vi "RT Driver VI.vi"(6 "Device Clock":string, 9 "Device Inputs FIFO":refnum<k33>, 10 "Device Outputs FIFO":refnum<k33>, 11 "Device Reference":T1 format="%.0x") -> ()   [LabVIEW 2020, in "Routing and Faulting Engine.lvlib"]
uses:
  Routing and Faulting Engine.lvlib
  <vilib>/NI VeriStand/Custom Device API/Custom Device Item Ref.ctl
  <vilib>/NI VeriStand/Custom Device Tools/Custom Device Utility Library/Custom Device Utility Library.lvlib
  <vilib>/NI VeriStand/Custom Device API/Custom Device API.lvlib
panel:
  in  "Initialization Status Notifier":refnum<notifier>
  in  "Status Notifier":refnum<notifier>
  # "Custom Device Template\nv1.0"
  # "Use this template as a starting point for creating a custom device code module. The input controls shown here are specially named controls that the system will use to provide the device loop with data. The controls are not required for the device loop to run. For instance, if the device doesn't produce any output data, then you don't need the Device Outputs FIFO control. If you do use these controls, however, they need to have these exact names to be functional."
  # "The optional status notifier element is used to notify the RT engine of the last state of the custom device, and to indicate the device has completed execution. If this control is not used, a default No Error value is returned to the system when the device finishes execution.\n\nNote: This error state is not checked until the system shuts down. Use an output status channel to send more immediate status values to the system."
  # "This optional input can be used to send the VeriStand Engine the final status of the custom device initalization process. If this control exists on the custom device front panel, the VeriStand Engine will wait for a status update before starting up. If the custom device reports an error, that will abort the execution of the current configuration in the VeriStand Engine.\n\nThis control can be deleted if the custom device does not need to send the initialization status update."
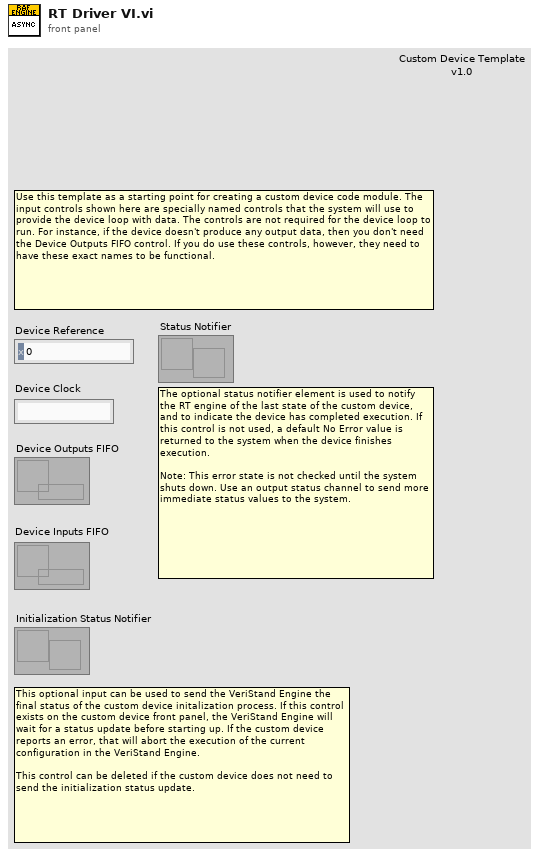
[diagram p1: front panel]
types:
  T1 = typedef "Custom Device API.lvlib/Custom Device Item Ref.ctl" = u64
  T2 = typedef "Custom Device API.lvlib/Custom Device Engine Event Ref.ctl" = refnum<event-registration>
  T3 = typedef "Routing and Faulting Engine.lvlib/Engine Data.ctl" = cluster{"Compiled.Settings":T4, "Producer":refnum<class "Abstract Producer.lvclass">, "Device Inputs":T13, "Device Outputs":T14, "States Changed":bool[]}
  T4 = typedef "Routing and Faulting Shared.lvlib/Compiled.Settings.ctl" = cluster{"Custom Device Name":string, "Communication Configuration":T5, "Routing and Faulting Configuration":T6, "Status Channels FIFO Indices":T12}
  T5 = typedef "Routing and Faulting Shared.lvlib/Communication Configuration.ctl" = cluster{"Consumer Queue Names":string[]}
  T6 = typedef "Routing and Faulting Shared.lvlib/Routing and Faulting Configuration.ctl" = cluster{"Routing Channel Configurations":T7[], "Alias Mappings":T9[], "Compiled Connection Buffer":T11[], "Compiled Initial Connection Indices":i32[]}
  T7 = typedef "Routing and Faulting Shared.lvlib/Routing Channel Configuration.ctl" = cluster{"Channel Name":string, "Initial Value":dbl, "FIFO Index":i32, "Value-Connections Map":T8}
  T8 = typedef "Routing and Faulting Shared.lvlib/Value-Connections Map.ctl" = cluster{"State Value Array":i32[], "Connection List Array":cluster{"Compiled Connections Indices":i32[]}[]}
  T9 = typedef "Routing and Faulting Shared.lvlib/Alias Mapping.ctl" = cluster{"Alias":string, "Endpoint":T10}
  T10 = typedef "Routing and Faulting Shared.lvlib/Alias Endpoint.ctl" = cluster{"Module Path":string, "Endpoint":string}
  T11 = typedef "Routing and Faulting Shared.lvlib/Compiled Connection.ctl" = cluster{"Consumer Queue Index":i32, "Normalized Connection String":string}
  T12 = typedef "Routing and Faulting Shared.lvlib/FIFO Indices.ctl" = cluster{"Status Channel":i32, "Heartbeat Channel":i32}
  T13 = typedef "Routing and Faulting Engine.lvlib/Device Inputs.ctl" = cluster{"Current Inputs":dbl[], "Previous Inputs":dbl[], "Device Inputs FIFO":refnum<k33>}
  T14 = typedef "Routing and Faulting Engine.lvlib/Device Outputs.ctl" = cluster{"Outputs":dbl[], "Device Outputs FIFO":refnum<k33>}
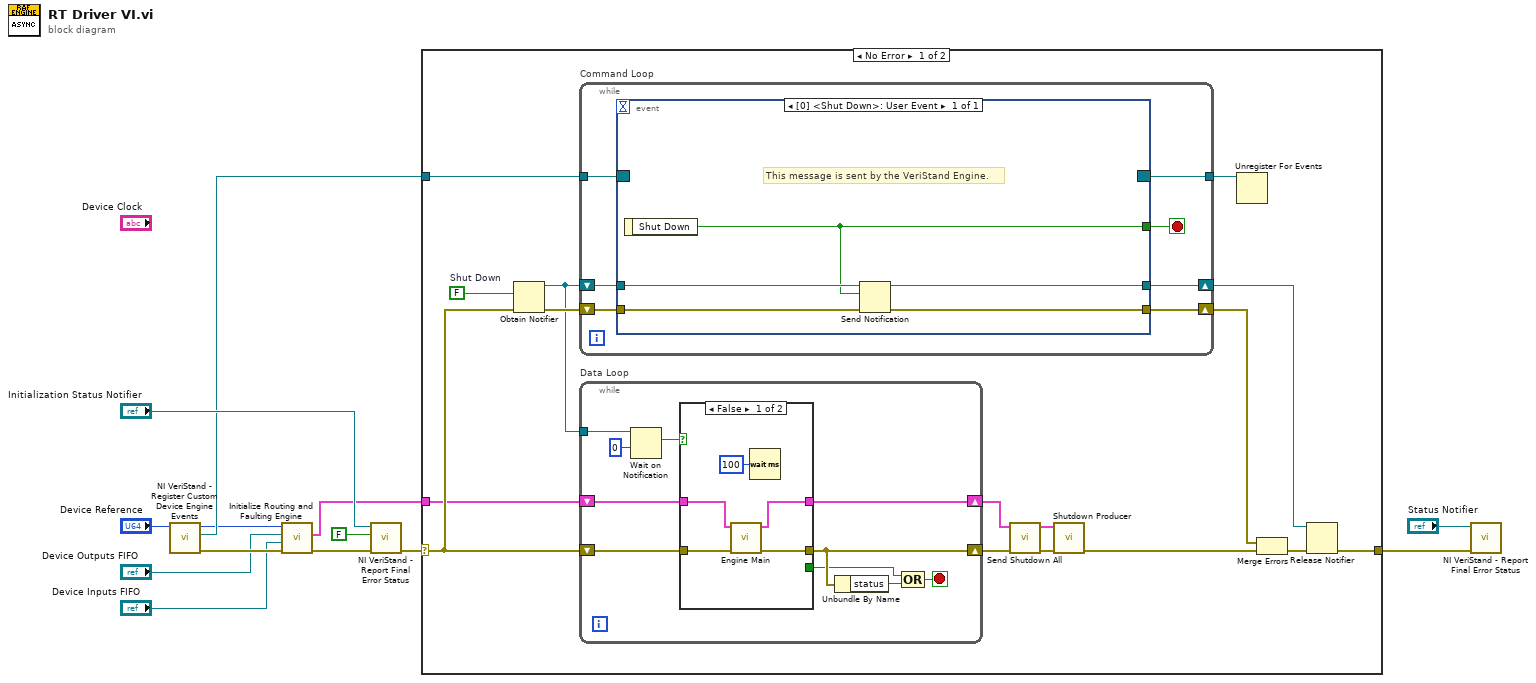
[diagram p0: block diagram]
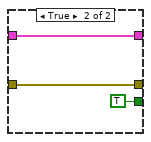
[diagram p2: hidden frame]
diagram:
  n1 = call <vilib>:"NI VeriStand - Register Custom Device Engine Events.vi"("Device Ref in"="Device Reference") -> ("error out"=w6:errorcluster, "Custom Device Engine Event Ref"=w11:T2, "Device Ref out"=w5:T1)  [unwired: 8 in]
  n2 = call "Initialize Routing and Faulting Engine.vi"("error in (no error)"=w6, "Device Inputs FIFO"="Device Inputs FIFO", "Device Outputs FIFO"="Device Outputs FIFO", "Device Ref in"=w5) -> ("error out"=w2:errorcluster, "Engine Data"=w1:T3)  [unwired: 5 in, 1 out]
  n3 = call <vilib>:"NI VeriStand - Report Final Error Status.vi"("error in (no error)"=w2, "Filter FIFO & Shutdown Errors (T)"=FALSE ("Filter FIFO Errors (T)"), "Status Notifier"="Initialization Status Notifier") -> ("error out"=w9:errorcluster)  [unwired: 8 out]
  n4 = case shown="No Error" w9 {
    selector: w9 -> [w22 w60]
    tunnel: w11 -> [w28 _]
    tunnel: [w26 w60] -> w10
    tunnel: w1 -> [w19 _]
    frame No Error {
      w27 = FALSE  # Shut Down
      n5 = Obtain Notifier(notification data type=w27, error in (no error)=w22) -> (notifier out=w24:refnum<notifier>, error out=w29:errorcluster)  [unwired: 2 in, 1 out]
      n6 = while "Command Loop" {
        tunnel: w28 -> [w36]
        tunnel: [w35] -> w25
        shift-right: [w32] -> w23
        shift-left: w24 -> [w33]
        shift-right: [w30] -> w20
        shift-left: w29 -> [w31]
        stop <- w34 stop-if-true
        n7 = event shown="[0] <Shut Down>: User Event" {
          selector: w36 -> [_]
          dyn-events: [_] -> w35
          timeout: _ -> [_]
          tunnel: [w39] -> w34
          tunnel: w33 -> [w40]
          tunnel: [w41] -> w32
          tunnel: w31 -> [w38]
          tunnel: [w37] -> w30
          event User Event {
            # "This message is sent by the VeriStand Engine."
            n8 = event-data() -> ("Shut Down"=w39:bool)  [unwired: 1 in]
            n9 = Send Notification(notification=w39, notifier=w40, error in (no error)=w38) -> (notifier out=w41:refnum<notifier>, error out=w37:errorcluster)
          }
        }
      }
      n10 = while "Data Loop" {
        shift-right: [w49] -> w14
        shift-left: w22 -> [w51]
        shift-right: [w42] -> w15
        shift-left: w19 -> [w43]
        tunnel: w24 -> [w48]
        stop <- w44 stop-if-true
        n11 = Wait on Notification(notifier=w48, timeout in ms (-1)=0) -> (notification=w47:bool)  [unwired: 2 in, 3 out]
        n12 = case shown="False" w47 {
          tunnel: w51 -> [w55 w58]
          tunnel: [w54 w58] -> w49
          tunnel: [_ TRUE] -> w45
          tunnel: w43 -> [w53 w57]
          tunnel: [w52 w57] -> w42
          frame False {
            n13 = call "Engine Main.vi"("error in (no error)"=w55, "Engine Data in"=w53) -> ("error out"=w54:errorcluster, "Engine Data out"=w52:T3)  [unwired: 8 in]
            n14 = Wait (ms)(milliseconds to wait=u32 100) -> ()  [unwired: 1 out]
          }
          frame True {
          }
        }
        n15 = Unbundle By Name(w49) -> ("status"=w46:bool)
        n16 = Compound Arithmetic op=OR(w45, w46) -> (w44:bool)
      }
      n17 = call "Send Shutdown All.vi"("error in (no error)"=w14, "Engine Data in"=w15) -> ("error out"=w17:errorcluster, "Engine Data out"=w16:T3)  [unwired: 8 in]
      n18 = call "Shutdown Producer.vi"("error in (no error)"=w17, "Engine Data in"=w16) -> ("error out"=w18:errorcluster)  [unwired: 8 in, 1 out]
      n19 = Unregister For Events(event registration refnum=w25) -> ()  [unwired: 1 in, 1 out]
      n20 = Merge Errors(w20, w18) -> (w21:errorcluster)
      n21 = Release Notifier(notifier=w23, error in (no error)=w21) -> (error out=w26:errorcluster)  [unwired: 1 in, 2 out]
    }
    frame Error {
    }
  }
  n22 = call <vilib>:"NI VeriStand - Report Final Error Status.vi"("error in (no error)"=w10, "Status Notifier"="Status Notifier") -> ()  [unwired: 1 in, 9 out]
